vi "test_ReservationWithEmptySessionInConnectionMap_CallGetConnectionsFromPinsForAllDcPowerPinsAllSites_ReturnsThreeConnections.vi"(8 "error in":errorcluster) -> (0 "error out":errorcluster, 2 "result":string, 3 "pass":bool)   [LabVIEW 2020, in "MeasurementServerTests.lvlib"]
uses:
  MeasurementServerTests.lvlib
  Runtime/Measurement Plugin Session Management V1/Session Reservation/Connection.ctl
  Runtime/Measurement Plugin Session Management V1/Session Reservation/Session Reservation.lvclass
  Runtime/Measurement Plugin Session Management V1/Session Reservation/Connection with Session.ctl
  c3cb69a0-23cd-49fc-99d1-8c54773f0200.vi
  Runtime/Sessions/niDCPower Sessions/Session Factory/Session Factory.lvclass
  Runtime/Measurement Plugin Session Management V1/Session Reservation/Pin Type.ctl
  4853e611-094c-40f3-9b92-adb7083f6e65.vi
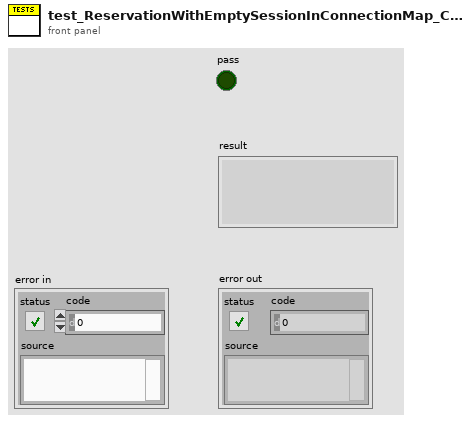
[diagram p1: front panel]
types:
  T1 = typedef "Measurement Plugin Session Management V1.lvlib/Session Reservation.lvclass/Pin Type.ctl" = enum16{"DUT and System Pins", "System Pins"}
  T2 = typedef "Measurement Plugin Session Management V1.lvlib/Session Reservation.lvclass/Connection with Session.ctl" = cluster{"connection":T3, "session":variant}
  T3 = typedef "Measurement Plugin Session Management V1.lvlib/Session Reservation.lvclass/Connection.ctl" = cluster{"pin or relay name":string, "site":i32, "instrument type id":string, "channel":string}
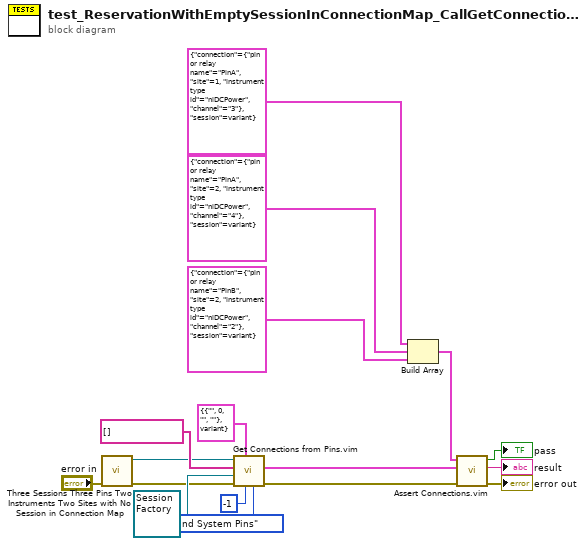
[diagram p0: block diagram]
diagram:
  n1 = call "Three Sessions Three Pins Two Instruments Two Sites with No Session in Connection Map.vi"("error in"="error in") -> ("error out"=w4:errorcluster, "session reservation out"=w3:refnum<class "Session Reservation.lvclass">)  [unwired: 9 in]
  n2 = call "Get Connections from Pins.vim"("pin type"=Pin_Type."DUT and System Pins", "site"=-1, "connection type"=T2 {"connection"={"pin or relay name"="", "site"=0, "instrument type id"="", "channel"=""}, "session"=variant} ("connection"), "error in"=w4, "session factory"=refnum<class "Session Factory.lvclass"> refnum ("MeasurementLink niDCPower.lvlib:Instrument.lvclass"), "pin or relay names"=string[] [], "session reservation in"=w3) -> ("error out"=w2:errorcluster, "connections"=w15:T2[])  [unwired: 2 in, 1 out]
  n3 = Build Array(T2 {"connection"={"pin or relay name"="PinA", "site"=1, "instrument type id"="niDCPower", "channel"="3"}, "session"=variant} ("connection out"), T2 {"connection"={"pin or relay name"="PinA", "site"=2, "instrument type id"="niDCPower", "channel"="4"}, "session"=variant} ("connection out"), T2 {"connection"={"pin or relay name"="PinB", "site"=2, "instrument type id"="niDCPower", "channel"="2"}, "session"=variant} ("connection out")) -> (w11:T2[])
  n4 = call "Assert Connections.vim"("error in"=w2, "actual connections"=w15, "expected connections"=w11) -> ("error out"=→"error out":errorcluster, "result"=→"result":string, "pass"=→"pass":bool)  [unwired: 6 in]
